vi "Boonton_get_GPIB-code_example.vi"() -> ()   [LabVIEW 2015]
uses:
  Hardware libraries/Boonton7200/Boonton7200_IEEE-488_Bus_Mnemonics.ctl
  Hardware libraries/Boonton7200/Boonton7200_Special_Function_Codes.ctl
  Hardware libraries/Boonton7200/Boonton7200.lvlib
panel:
  out "GPIB code":string
  in  "Special Functions":T1
  in  "Data Value":sgl
  in  "IEEE-488 Bus Mnemonics":T2
  out "Error Out":errorcluster
  in  "Error In":errorcluster
  in  "Stop Button":bool
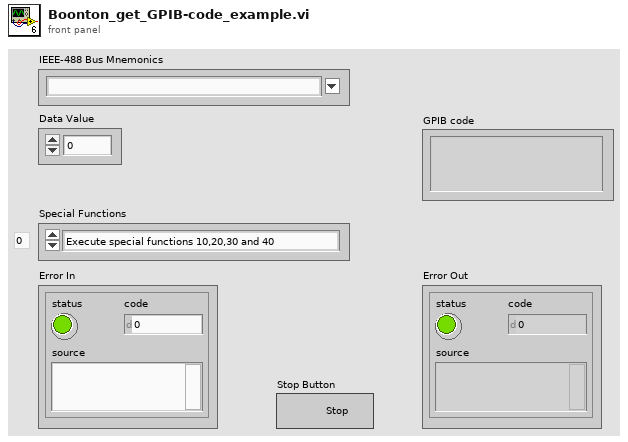
[diagram p1: front panel]
types:
  T1 = typedef "Boonton7200_Special_Function_Codes.ctl" = enum16{"Execute special functions 10,20,30 and 40", "Test Level display and entry", "Capacitance Standard display and entry", "Conductance Standard dispaly and entry", "Capacitance Low Limit display and entry", "Capacitance High Limit dispaly and entry", "IEEE-488 Bus Address display and entry", "End-of-string charecter display and selection", "Capacitance uncertainty display", "Conductance uncertainty dispaly", "Automatic selection(Measurement Ranging Functions)", "Hold current measurement range", "Set and hold 2.000 pF / 2.00 uS range", "Set and hold 20.00 pF / 20.0 uS range", "Set and hold 200.0 pF / 200 uS range", "Set and holde 2000 pF / 2000 uS range", "16 - Not Defined", "17 - Not Defined", "18 - Not Defined", "19 - Not Defined", "Automatic selection(Internal Bias Ranging Functions)", "Hold current bias range", "Set and hold 20.000 V range", "Set and Hold 100.00 V range", "24 - Not Defined", "25 - Not Defined", "26 - Not Defined", "27 - Not Defined", "28 - Not Defined", "29 - Not Defined", "30 Automatic selection(Measurement Filter Functions)", "Filter length = 1 measurement, no average", "Filter length = 2 measurement", "Filter length = 5 measurement", "Filter length = 10 measurement", "Filter length = 20 measurement", "Filter length = 50 measurement", "Filter length = 100 measurement", "Filter length = 200 measurement", "Filter length = 500 measurement", "Normal operation, free-run dispaly(Sercvice Request Functions)", "Disable SRQ interrupt", "Enable SRQ interrupt", "Set SRQ mask when an error occurs", "Set SRQ mask and update dispaly when measurement filter is complete", "Set SRQ mask when capacitance measurement is within the high and low limit settings", "Set SRQ mask when capacitance measurement exceeds the high or low limit settings", "Set SRQ mask when zero or calibration is complete", "Set SRQ mask when sweep is complete", "49 - Not Defined", "Calibrate detector offset(Automatic Calibration and Test Functions)", "Calibrate external bias offset", "Calibrate internal bias offset", "Calibrate full-scale capacitance", "Calibrate conductance phase", "Display internal temperature", "Display amplitude error due to temperature influence", "Display phase error due to temperature influence", "Initialize instrument and erase all program locations", "Initalize software calibration variables"}
  T2 = typedef "Boonton7200_IEEE-488_Bus_Mnemonics.ctl" = string
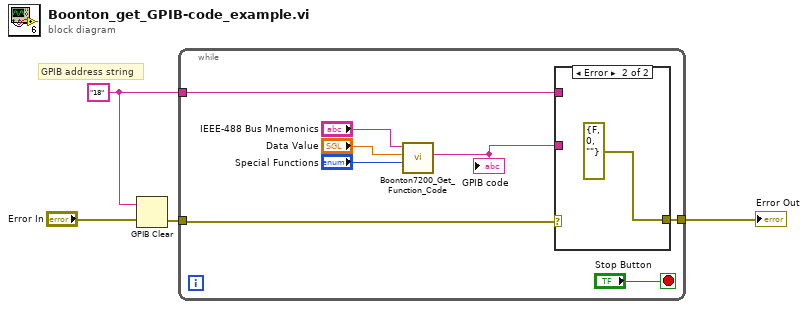
[diagram p0: block diagram]
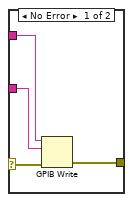
[diagram p2: hidden frame]
diagram:
  w3 = "18" ("address string")
  # "GPIB address string"
  n1 = GPIB Clear(2:"Error In", 3:w3) -> (0:w4:errorcluster)  [unwired: 1 out]
  n2 = while {
    tunnel: w4 -> [w8]
    tunnel: w3 -> [w6]
    tunnel: [w7] -> w1
    stop <- "Stop Button" stop-if-true
    n3 = call "Boonton7200_Get_Function_Code.vi"("Special Functions"="Special Functions", "Data Value"="Data Value", "IEEE-488 Bus Mnemonics"="IEEE-488 Bus Mnemonics") -> ("GPIB code (IEEE-488)"=w5:string)  [unwired: 7 in, 1 out]
    "GPIB code" <- w5
    n4 = case shown="Error" w8 {
      selector: w8 -> [w16 _]
      tunnel: [w15 errorcluster {"status"=FALSE, "code"=0, "source"=""} ("error constant")] -> w7
      tunnel: w6 -> [w14 _]
      tunnel: w5 -> [w13 _]
      frame No Error {
        n5 = GPIB Write(0:w14, 1:w13, 3:w16) -> (6:w15:errorcluster)  [unwired: 2 in, 1 out]
      }
      frame Error {
      }
    }
  }
  "Error Out" <- w1
